vi "Write Price Data RealTime DVR.vi"(8 "error in":errorcluster, 10 "PriceData_RealTime":T1, 11 "EMS Generic in":refnum<class "EMS Generic.lvclass">) -> (0 "error out":errorcluster, 3 "EMS Generic out":refnum<class "EMS Generic.lvclass">)   [LabVIEW 2018, in "EMS Generic Actor.lvlib" / "EMS Generic.lvclass"]
uses:
  EMS Generic.lvclass
  <vilib>/ORNL/CSEISMIC DDS/CSEISMIC DDS Base/Data Types/PriceData_RealTime.ctl
  <vilib>/ORNL/CSEISMIC DDS/CSEISMIC DDS Base/Data Types/Controls/DeviceID.ctl
  EMS Generic.lvclass/EMS Generic.ctl
  <vilib>/ORNL/CSEISMIC DDS/CSEISMIC DDS Base/CSEISMIC DDS.lvclass
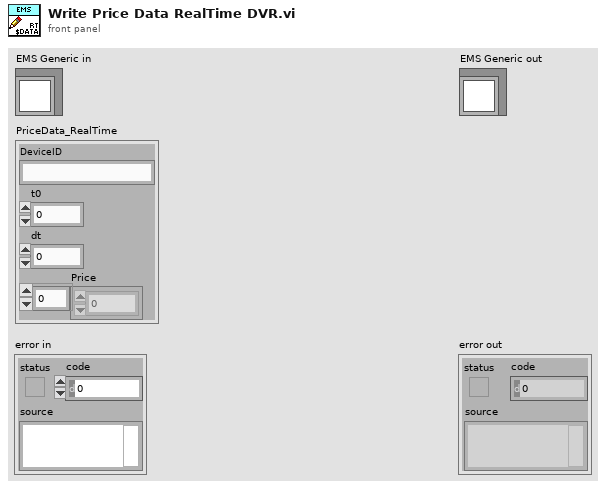
[diagram p1: front panel]
types:
  T1 = typedef "CSEISMIC DDS.lvlib/CSEISMIC DDS.lvclass/PriceData_RealTime.ctl" = cluster{"DeviceID":T2, "t0":dbl, "dt":dbl, "Price":dbl[]}
  T2 = typedef "CSEISMIC DDS.lvlib/CSEISMIC DDS.lvclass/DeviceID.ctl" = string
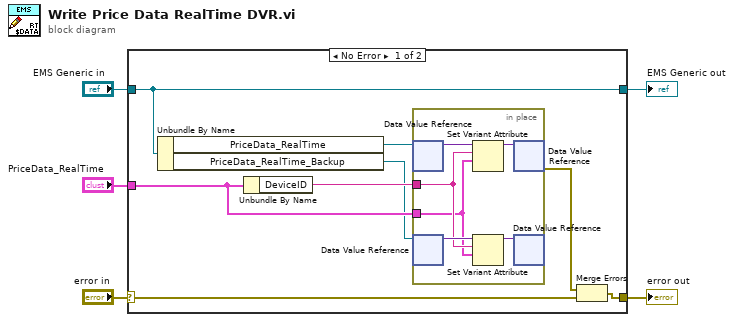
[diagram p0: block diagram]
diagram:
  n1 = case shown="No Error" "error in" {
    selector: "error in" -> [w13 w21]
    tunnel: [w8 w21] -> w4
    tunnel: [w12 w20] -> w2
    tunnel: "EMS Generic in" -> [w12 w20]
    tunnel: "PriceData_RealTime" -> [w10 _]
    frame No Error {
      n2 = Unbundle By Name(w12) -> ("PriceData_RealTime"=w9:refnum<data-value>, "PriceData_RealTime_Backup"=w6:refnum<data-value>)
      n3 = Unbundle By Name(w10) -> ("DeviceID"=w11:T2)
      n4 = in-place {
        in-place-border: w11 -> [w15]
        in-place-border: w10 -> [w14]
        n5 = in-place-dvr #1(w9) -> (w19:variant)  [unwired: 1 out]
        n6 = in-place-dvr #2(w6) -> (w17:variant)  [unwired: 1 out]
        n7 = Set Variant Attribute(Variant=w19, name=w15, value=w14) -> (Variant out=w18:variant)  [unwired: 1 in, 2 out]
        n8 = Set Variant Attribute(Variant=w17, name=w15, value=w14) -> (Variant out=w16:variant)  [unwired: 1 in, 2 out]
        n9 = in-place-dvr #1(w18) -> (w7:errorcluster)  [unwired: 1 out]
        n10 = in-place-dvr #2(w16) -> ()  [unwired: 2 out]
      }
      n11 = Merge Errors(w7, w13) -> (w8:errorcluster)
    }
    frame Error {
    }
  }
  "error out" <- w4
  "EMS Generic out" <- w2
